vi "FTW-Endpoint-Multipart-Tell.vi"(0 "FTW ØMQ Endpoint":refnum<class "FTW-Endpoint-ZMQ.lvclass">, 5 "Multipart Message":string[](array[string]), 7 "Timeout":i32 format="%dmsec", 11 "error in":errorcluster) -> (4 "FTW ØMQ Endpoint out":refnum<class "FTW-Endpoint-ZMQ.lvclass">, 8 "Timed out?":bool, 15 "error out":errorcluster)   [LabVIEW 2012, in "FTW-Actor.lvlib" / "FTW-Endpoint-ZMQ.lvclass"]
uses:
  FTW-Endpoint-ZMQ.lvclass
  FTW-Endpoint-ZMQ.lvclass/FTW-Endpoint-ZMQ.ctl
  FTW-ZMQ-LibraryFilepath.vi
  FTW-ZMQ-LibraryReturnValue.vi
panel:
  # "Inputs"
  # "Outputs"
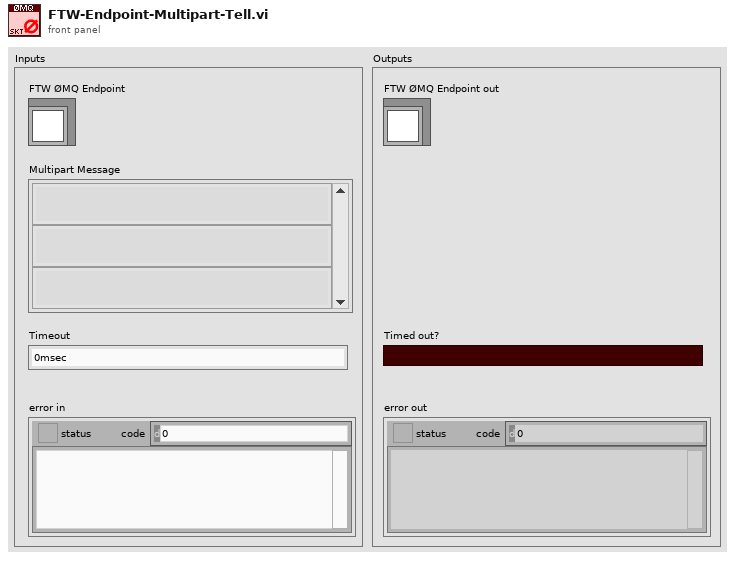
[diagram p1: front panel]
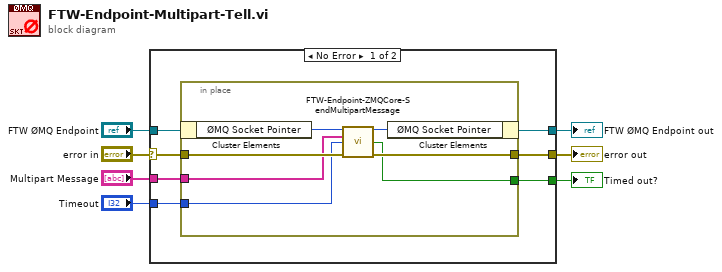
[diagram p0: block diagram]
diagram:
  n1 = case shown="No Error" "error in" {
    selector: "error in" -> [w10 w22]
    tunnel: "FTW ØMQ Endpoint" -> [w14 w23]
    tunnel: "Multipart Message" -> [w13 _]
    tunnel: [w12 w22] -> w5
    tunnel: [w11 w23] -> w4
    tunnel: "Timeout" -> [w9 _]
    tunnel: [w8 _] -> w1
    frame No Error {
      n2 = in-place {
        in-place-border: w13 -> [w17]
        in-place-border: w10 -> [w21]
        in-place-border: [w20] -> w12
        in-place-border: w9 -> [w16]
        in-place-border: [w15] -> w8
        n3 = in-place-cluster #1(w14) -> ("ØMQ Socket Pointer"=w19:u64)
        n4 = call "FTW-Endpoint-ZMQCore-SendMultipartMessage.vi"("ØMQ Socket Pointer"=w19, "Multipart Message"=w17, "Write Timeout"=w16, "error in"=w21) -> ("ØMQ Socket Pointer out"=w18:u64, "Write Timed out?"=w15:bool, "error out"=w20:errorcluster)  [unwired: 9 in]
        n5 = in-place-cluster #1("ØMQ Socket Pointer"=w18) -> (w11:refnum<class "FTW-Endpoint-ZMQ.lvclass">)
      }
    }
    frame Error {
    }
  }
  "error out" <- w5
  "FTW ØMQ Endpoint out" <- w4
  "Timed out?" <- w1
